vi "FGV T90.vi"(0 "T90 Konfig Daten":T3={"Bearbeiter:"="", "Komponente:"=0, "Gasflaschen Nr.:"="", "Accuracy"=0.0, "Sollwert"=0.0, "Modus"=0, "Abschaltzeit:"=120.0, "Abweichung:"=3.0, "Pfad:"=path "D:/IAG_Data/Log", "Textname:"="", "CG Aufschaltzeit:"=120.0, "Einheit"="", "N2 Aufschaltzeit:"=120.0, "Analysator"="", "Gasflasche"=0, "Konfig Gasflasche"=FALSE, "Frequency:"=0} {"Frequency:" items=["5 Hz"=5, "10 Hz"=10]; "Gasflasche" items=["----"=10000, "IAG NH3 3000"=0, "IAG NH3 200"=1, "IAG NH3 2000"=2, "IAG MG"=3, "IAG O2"=4]; "N2 Aufschaltzeit:" min=30.0; "CG Aufschaltzeit:" min=60.0; "Abweichung:" min=2.0; "Abschaltzeit:" min=60.0; "Modus" items=["CG zu PNS", "CG zu Entnahmestelle"]}, 11 "error in (no error)":errorcluster caption="Fehler (Eingang, kein Fehler)", 12 "Result Textfile":T1, 13 "Aktion":T9) -> (4 "T90 Konfig Daten":T3={"Bearbeiter:"="", "Komponente:"=0, "Gasflaschen Nr.:"="", "Accuracy"=0.0, "Sollwert"=0.0, "Modus"=0, "Abschaltzeit:"=120.0, "Abweichung:"=3.0, "Pfad:"=path "D:/IAG_Data/Log", "Textname:"="", "CG Aufschaltzeit:"=120.0, "Einheit"="", "N2 Aufschaltzeit:"=120.0, "Analysator"="", "Gasflasche"=0, "Konfig Gasflasche"=FALSE, "Frequency:"=0} {"Frequency:" items=["5 Hz"=5, "10 Hz"=10]; "Gasflasche" items=["----"=10000, "IAG NH3 3000"=0, "IAG NH3 200"=1, "IAG NH3 2000"=2, "IAG MG"=3, "IAG O2"=4]; "N2 Aufschaltzeit:" min=30.0; "CG Aufschaltzeit:" min=60.0; "Abweichung:" min=2.0; "Abschaltzeit:" min=60.0; "Modus" items=["CG zu PNS", "CG zu Entnahmestelle"]}, 6 "T90 Aktiv":bool, 8 "Ext. Ventil aktiv":bool, 10 "N2 spülen aktiv":bool, 14 "Result Textfile":T1, 15 "error out":errorcluster caption="Fehler (Ausgang)")   [LabVIEW 2020, in "EPA 1065.lvlib" / "T90 Test 1065-308.lvlib"]
uses:
  T90 Test 1065-308.lvlib
  Aktion FGV T90.ctl
  T90 Konfig Daten.ctl
  Modus.ctl
  Seiten/System Einstellungen V2/Analysatoren.ctl
  Seiten/System Einstellungen V2/Gasflasche Auswahl.ctl
  Seiten/System Einstellungen V2/Konfig Gasflasche.ctl
  Frequenz.ctl
  Result Textfile.ctl
  Ergebnis.ctl
  Seiten/CalGas Aufschaltung/FGV CalGas Aktionen.ctl
  Seiten/CalGas Aufschaltung/Auswahl Aufschaltpunkt.ctl
  Allgemein/allgemeine Sub-VIs.lvlib
  Seiten/CalGas Aufschaltung/CalGas Aufschaltung.lvlib
  Seiten/System Einstellungen V2/System Einstellungen V2.lvlib
panel:
  # "sec."
  # "sec."
  # "%"
  # "%"
  # "sec."
  # "sec."
  # "sec."
  # "%"
  # "%"
  # "sec."
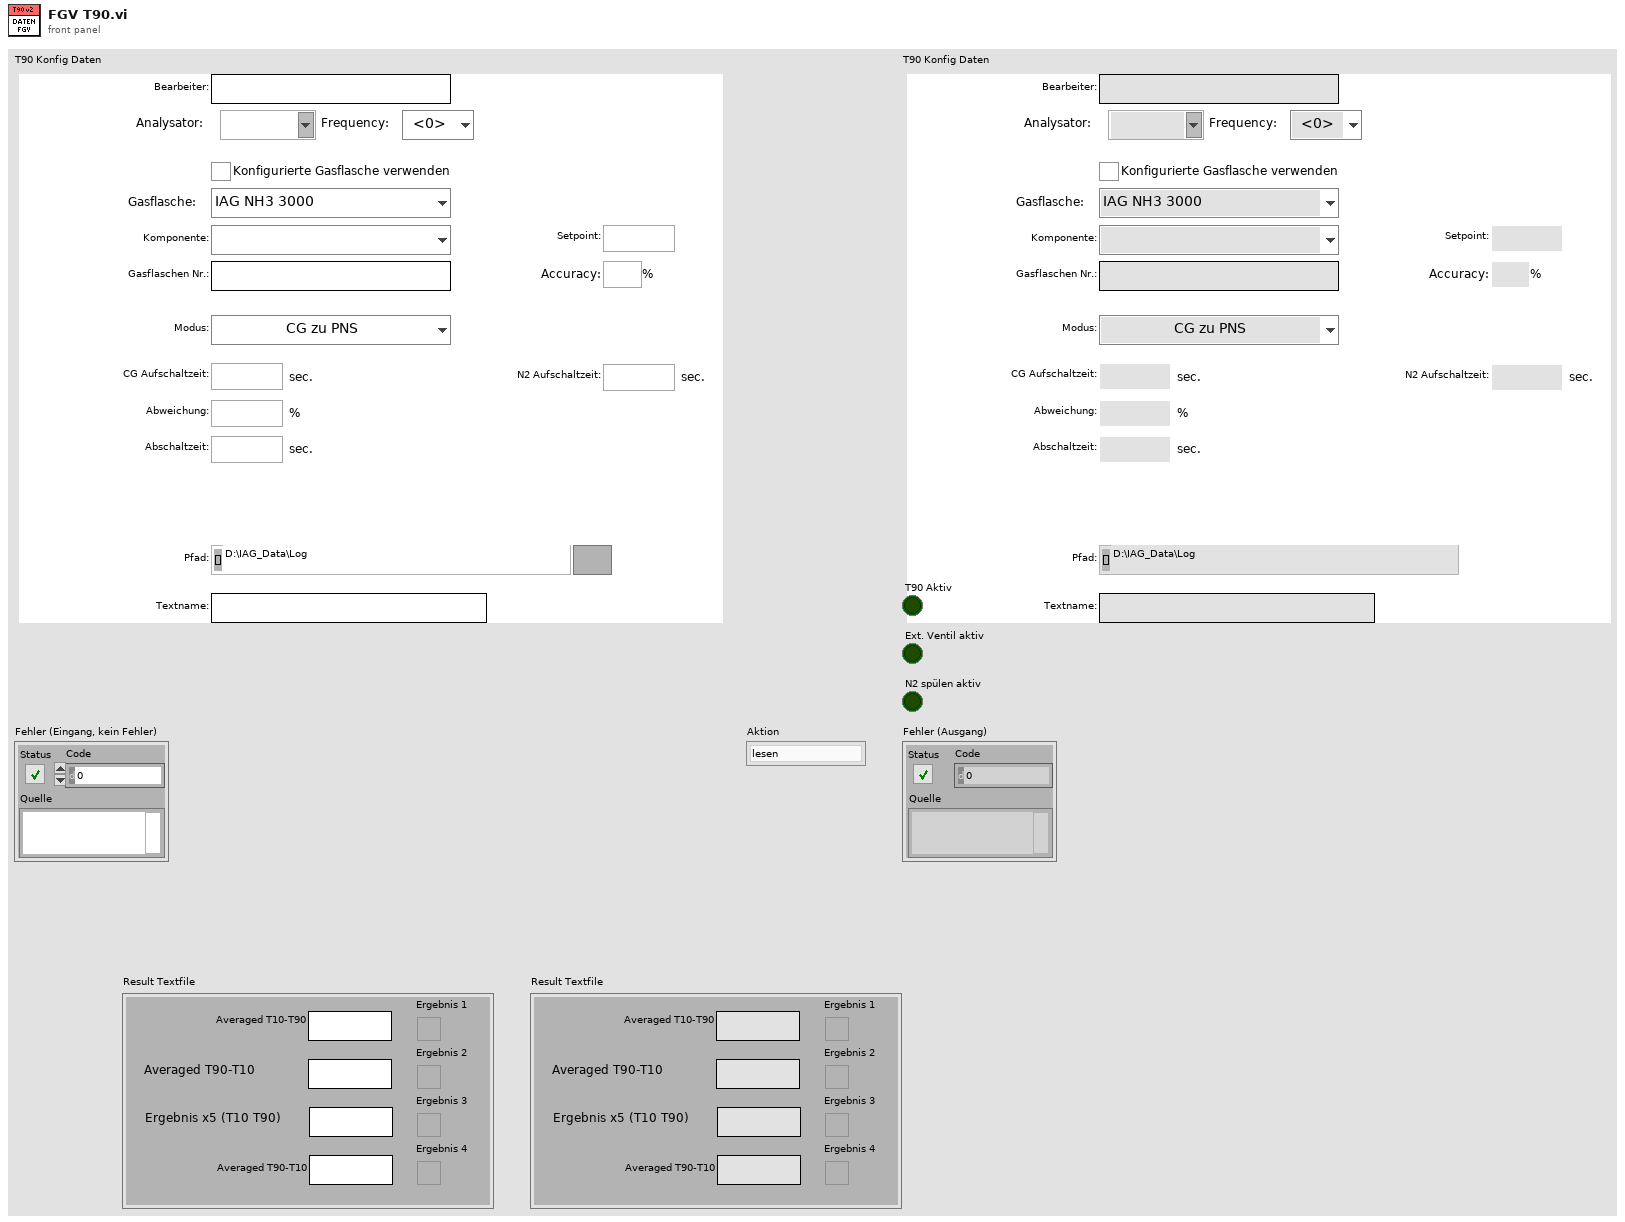
[diagram p1: front panel]
types:
  T1 = typedef "EPA 1065.lvlib/T90 Test 1065-308.lvlib/Result Textfile.ctl" = cluster{"Averaged T10-T90":string, "Averaged T90-T10":string, "Ergebnis x5 (T10 T90)":string, "Ergebnis x5 (T90 T10)":string, "Ergebnis 1":T2, "Ergebnis 2":T2, "Ergebnis 3":T2, "Ergebnis 4":T2}
  T2 = typedef "EPA 1065.lvlib/T90 Test 1065-308.lvlib/Ergebnis.ctl" = bool
  T3 = typedef "EPA 1065.lvlib/T90 Test 1065-308.lvlib/T90 Konfig Daten.ctl" = cluster{"Bearbeiter:":string, "Komponente:":u16, "Gasflaschen Nr.:":string, "Accuracy":dbl, "Sollwert":dbl, "Modus":T4, "Abschaltzeit:":dbl, "Abweichung:":dbl, "Pfad:":path, "Textname:":string, "CG Aufschaltzeit:":dbl, "Einheit":string, "N2 Aufschaltzeit:":dbl, "Analysator":T5, "Gasflasche":T6, "Konfig Gasflasche":T7, "Frequency:":T8}
  T4 = typedef "EPA 1065.lvlib/T90 Test 1065-308.lvlib/Modus.ctl" = u16
  T5 = typedef "System Einstellungen V2.lvlib/Analysatoren.ctl" = string
  T6 = typedef "System Einstellungen V2.lvlib/Gasflasche Auswahl.ctl" = u16
  T7 = typedef "System Einstellungen V2.lvlib/Konfig Gasflasche.ctl" = bool
  T8 = typedef "EPA 1065.lvlib/T90 Test 1065-308.lvlib/Frequenz.ctl" = u16
  T9 = typedef "EPA 1065.lvlib/T90 Test 1065-308.lvlib/Aktion FGV T90.ctl" = enum16{"lesen", "Konfig Daten", "speichern", "laden", "T90 aktiv", "T90 inaktiv", "Ext. Ventil aktivieren", "Ext. Ventil deaktivieren", "N2 spülen aktiv", "N2 spülen inaktiv", "Ergebnis Textfile"}
  T10 = enum16{"open", "replace", "create", "open or create", "replace or create", "replace or create with confirmation"}
  T11 = typedef "CalGas Aufschaltung.lvlib/Auswahl Aufschaltpunkt.ctl" = enum16{"über Filterblock", "Analysator direkt", "über PNS", "Entnahme", "Gasdivider"}
  T12 = typedef "CalGas Aufschaltung.lvlib/FGV CalGas Aktionen.ctl" = enum16{"lesen", "Analysator Auswahl", "Def.CalGas", "Aufschaltung CalGas", "laden", "speichern", "KAL extrahieren"}
  T13 = typedef "CalGas Aufschaltung.lvlib/Aufschaltung CalGas.ctl" = cluster{"Kalibriergas":T14, "Aufschaltpunkt":T11, "Analysator":T15}
  T14 = typedef "Auswahlfeld.ctl" = u16
  T15 = typedef "CalGas Aufschaltung.lvlib/Auswahl Analysator.ctl" = enum16{"FT-IR", "FID", "PMA", "PMA/FID/FT-IR"}
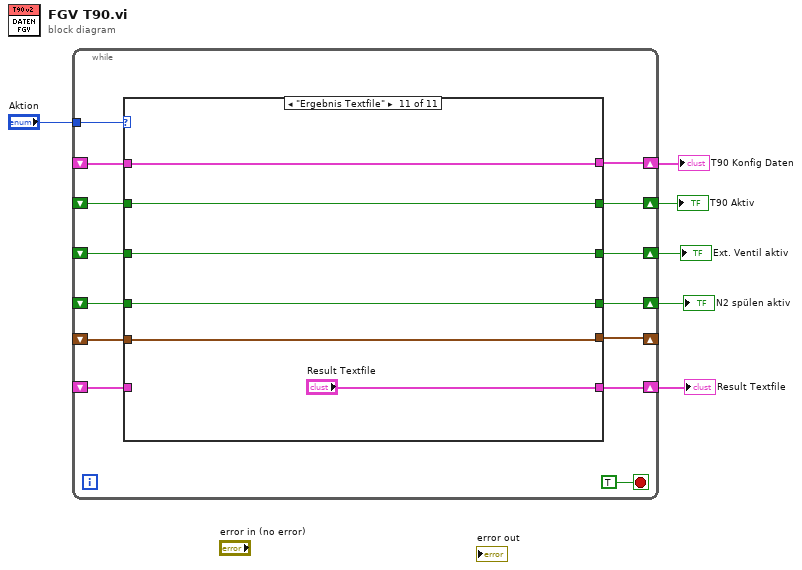
[diagram p0: block diagram]
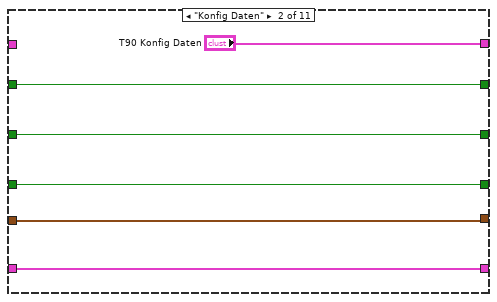
[diagram p3: hidden frame]
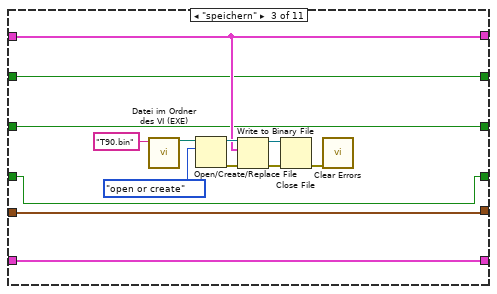
[diagram p4: hidden frame]
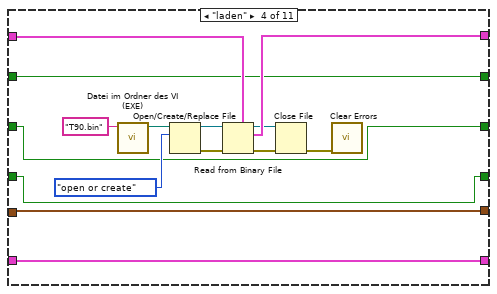
[diagram p5: hidden frame]
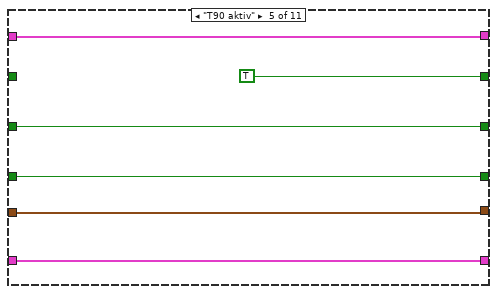
[diagram p6: hidden frame]
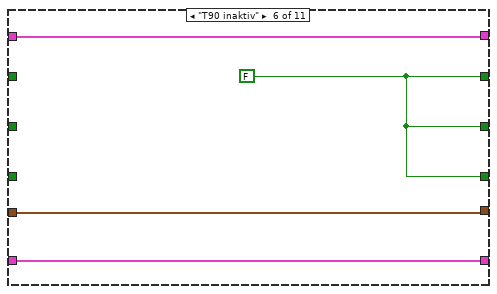
[diagram p7: hidden frame]
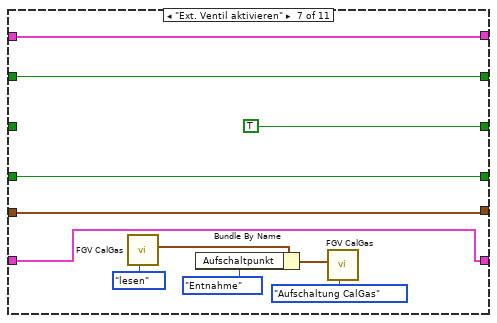
[diagram p8: hidden frame]
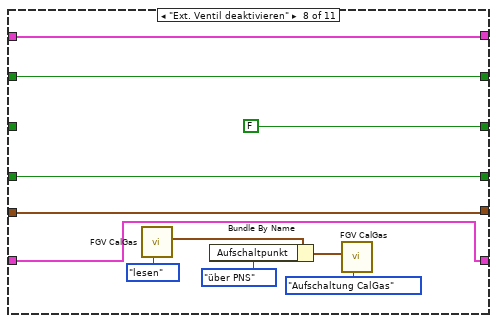
[diagram p9: hidden frame]
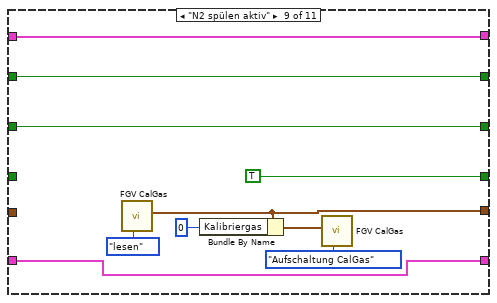
[diagram p10: hidden frame]
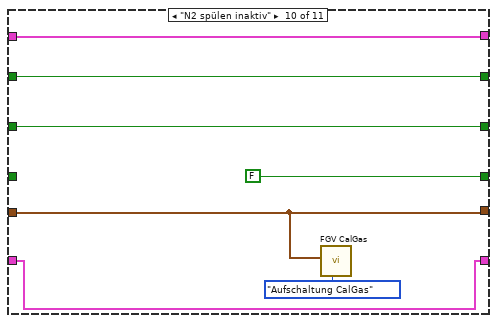
[diagram p11: hidden frame]
diagram:
  n1 = while {
    tunnel: "Aktion" -> [w20]
    shift-right: [w19] -> w5
    shift-left: _ -> [w18]
    shift-right: [w16] -> w4
    shift-left: _ -> [w15]
    shift-right: [w14] -> w3
    shift-left: _ -> [w13]
    shift-right: [w11] -> w2
    shift-left: _ -> [w12]
    shift-right: [w10] -> _
    shift-left: _ -> [w9]
    shift-right: [w8] -> w1
    shift-left: _ -> [w7]
    stop <- TRUE stop-if-true
    n2 = case shown="\"Ergebnis Textfile\"" w20 {
      tunnel: [w26 "T90 Konfig Daten" w39 w59 w67 w71 w82 w93 w103 w110 w116] -> w19
      tunnel: w18 -> [w26 _ w39 w60 w67 w71 w82 w93 w103 w110 w116]
      tunnel: [w25 w31 w37 w51 TRUE ("T90 Aktiv") w70 w80 w91 w100 w107 w115] -> w16
      tunnel: w15 -> [w25 w31 w37 w51 _ _ w80 w91 w100 w107 w115]
      tunnel: [w24 w30 w36 w50 w65 w70 TRUE ("T90 Aktiv") FALSE ("T90 Aktiv") w102 w109 w114] -> w14
      tunnel: w13 -> [w24 w30 w36 w50 w65 _ _ _ w102 w109 w114]
      tunnel: [w23 w29 w35 w49 w64 w70 w79 w90 TRUE ("T90 Aktiv") FALSE ("T90 Aktiv") w113] -> w11
      tunnel: w12 -> [w23 w29 w35 w49 w64 _ w79 w90 _ _ w113]
      tunnel: [w22 w28 w34 w48 w63 w69 w73 w84 w95 w105 w112] -> w10
      tunnel: w9 -> [w22 w28 w34 w48 w63 w69 w73 w84 _ w105 w112]
      tunnel: [w21 w27 w33 w47 w62 w68 w72 w83 w94 w104 "Result Textfile"] -> w8
      tunnel: w7 -> [w21 w27 w33 w47 w62 w68 w72 w83 w94 w104 _]
      frame "lesen", Default {
      }
      frame "Konfig Daten" {
      }
      frame "speichern" {
        n3 = call "Datei im Ordner des VI (EXE).vi"("Dateiname"="T90.bin") -> ("Dateipfad im Ordner des Haupt-VIs"=w41:path)  [unwired: 8 in, 2 out]
        n4 = Open/Create/Replace File(file path (use dialog)=w41, operation (0:open)=T10."open or create" ("Operation (0:open)")) -> (refnum out=w40:refnum<file>, error out=w42:errorcluster)  [unwired: 4 in, 1 out]
        n5 = Write to Binary File(file (use dialog)=w40, data=w39, error in=w42) -> (refnum out=w44:refnum<file>, error out=w45:errorcluster)  [unwired: 3 in, 1 out]
        n6 = Close File(refnum=w44, error in=w45) -> (error out=w38:errorcluster)  [unwired: 1 out]
        n7 = call <vilib>:"Clear Errors.vi"("error in (no error)"=w38) -> ()  [unwired: 5 in, 2 out]
      }
      frame "laden" {
        n8 = call "Datei im Ordner des VI (EXE).vi"("Dateiname"="T90.bin") -> ("Dateipfad im Ordner des Haupt-VIs"=w55:path)  [unwired: 8 in, 2 out]
        n9 = Open/Create/Replace File(file path (use dialog)=w55, operation (0:open)=T10."open or create" ("Operation (0:open)")) -> (refnum out=w53:refnum<file>, error out=w54:errorcluster)  [unwired: 4 in, 1 out]
        n10 = Read from Binary File(5:w60, 8:w54, 11:w53) -> (0:w58:errorcluster, 2:w59:T3, 3:w56:refnum<file>)  [unwired: 3 in, 1 out]
        n11 = Close File(refnum=w56, error in=w58) -> (error out=w57:errorcluster)  [unwired: 1 out]
        n12 = call <vilib>:"Clear Errors.vi"("error in (no error)"=w57) -> ()  [unwired: 5 in, 2 out]
      }
      frame "T90 aktiv" {
      }
      frame "T90 inaktiv" {
        w70 = FALSE ("T90 Aktiv")
      }
      frame "Ext. Ventil aktivieren" {
        n13 = call "FGV CalGas.vi"("Aktionen"=FGV_CalGas_Aktionen."lesen") -> ("Aufschaltung CalGas"=w76:T13)  [unwired: 6 in, 4 out]
        n14 = Bundle By Name(cluster=w76, "Aufschaltpunkt"=Auswahl_Aufschaltpunkt."Entnahme") -> (w74:T13)
        n15 = call "FGV CalGas.vi"("Aktionen"=FGV_CalGas_Aktionen."Aufschaltung CalGas", "Aufschaltung CalGas"=w74) -> ()  [unwired: 5 in, 5 out]
      }
      frame "Ext. Ventil deaktivieren" {
        n16 = call "FGV CalGas.vi"("Aktionen"=FGV_CalGas_Aktionen."lesen") -> ("Aufschaltung CalGas"=w87:T13)  [unwired: 6 in, 4 out]
        n17 = Bundle By Name(cluster=w87, "Aufschaltpunkt"=Auswahl_Aufschaltpunkt."über PNS") -> (w85:T13)
        n18 = call "FGV CalGas.vi"("Aktionen"=FGV_CalGas_Aktionen."Aufschaltung CalGas", "Aufschaltung CalGas"=w85) -> ()  [unwired: 5 in, 5 out]
      }
      frame "N2 spülen aktiv" {
        n19 = call "FGV CalGas.vi"("Aktionen"=FGV_CalGas_Aktionen."lesen") -> ("Aufschaltung CalGas"=w95:T13)  [unwired: 6 in, 4 out]
        n20 = Bundle By Name(cluster=w95, "Kalibriergas"=0) -> (w97:T13)
        n21 = call "FGV CalGas.vi"("Aktionen"=FGV_CalGas_Aktionen."Aufschaltung CalGas", "Aufschaltung CalGas"=w97) -> ()  [unwired: 5 in, 5 out]
      }
      frame "N2 spülen inaktiv" {
        n22 = call "FGV CalGas.vi"("Aktionen"=FGV_CalGas_Aktionen."Aufschaltung CalGas", "Aufschaltung CalGas"=w105) -> ()  [unwired: 5 in, 5 out]
      }
      frame "Ergebnis Textfile" {
      }
    }
  }
  "T90 Konfig Daten" <- w5
  "T90 Aktiv" <- w4
  "Ext. Ventil aktiv" <- w3
  "N2 spülen aktiv" <- w2
  "Result Textfile" <- w1
